vi "ClimbAverages.vi"(0 "Number in":string, 1 "String in":string) -> (7 "String out":string, 8 "Number out":string)   [LabVIEW 2015]
panel:
  in  "Counter":i32
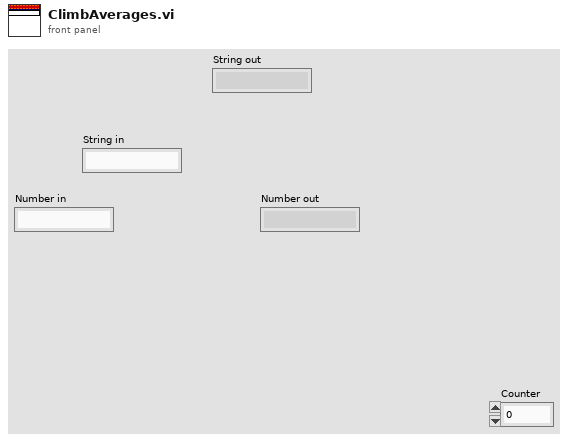
[diagram p1: front panel]
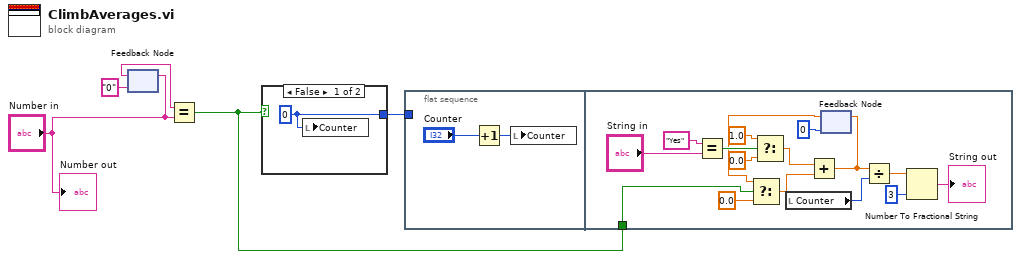
[diagram p0: block diagram]
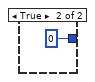
[diagram p2: hidden frame]
diagram:
  n1 = feedback #1("0" ("Number in")) -> (w3:string)
  n2 = feedback-in #1("Number in") -> ()
  n3 = Equal?(x=w3, y="Number in") -> (x = y?=w1:bool)
  n4 = case shown="False" w1 {
    tunnel: [w6 0 ("Counter")] -> w5
    frame False {
      w6 = 0 ("Counter")
      n5 = local write "Counter"(w6) -> ()
    }
    frame True {
    }
  }
  n6 = flat-sequence {
    tunnel: w5 -> [_]
    tunnel: w1 -> [w11]
    frame #0 {
      n7 = Increment(x="Counter") -> (x+1=w8:i32)
      n8 = local write "Counter"(w8) -> ()
    }
    frame #1 {
      n9 = Equal?(x="Yes", y="String in") -> (x = y?=w21:bool)
      n10 = Select(t=1.0, s=w21, f=0.0 ("t")) -> (s? t:f=w16:dbl)
      n11 = local read "Counter"() -> (w15:i32)
      n12 = feedback #2(0) -> (w14:dbl)
      n13 = Select(t=w14, s=w11, f=0.0) -> (s? t:f=w12:dbl)
      n14 = Add(x=w16, y=w12) -> (x+y=w24:dbl)
      n15 = feedback-in #2(w24) -> ()
      n16 = Divide(x=w24, y=w15) -> (x/y=w22:dbl)
      n17 = Number To Fractional String(number=w22, precision (6)=i16 3) -> (F-format string=→"String out":string)  [unwired: 2 in]
    }
  }
  "Number out" <- "Number in"
